vi "practica3.vi"() -> ()   [LabVIEW 2016]
uses:
  <vilib>/addons/Fuzzy Logic/NI_Fuzzy_Logic_API.lvlib
  <vilib>/addons/Fuzzy Logic/Membership/FL Create Membership Function (Trapezoid).vi
  <vilib>/addons/Fuzzy Logic/Membership/FL Create Membership Function (Triangle).vi
  <vilib>/addons/Fuzzy Logic/TypeDefs/FL Input_Output.ctl
  <vilib>/addons/Fuzzy Logic/TypeDefs/FL Modifier.ctl
panel:
  out "membership functions plot":cluster{cluster{"Xi":dbl, "Yi":dbl}[]}[](graph)
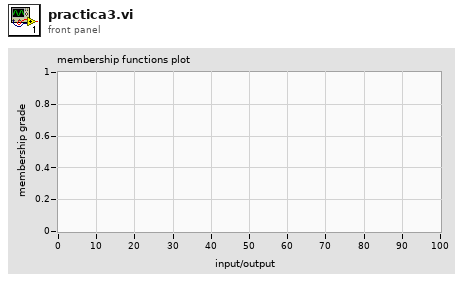
[diagram p1: front panel]
types:
  T1 = cluster{string, enum16{"triangular", "trapezoidal"}, dbl[]}[]
  T2 = typedef "NI_Fuzzy_Logic_API.lvlib/FL Input_Output.ctl" = u16
  T3 = typedef "NI_Fuzzy_Logic_API.lvlib/FL Modifier.ctl" = u16
  T4 = typedef "NI_Fuzzy_Logic_API.lvlib/FL Antecedent.ctl" = cluster{"Var Index":i32, "MF Index":i32, "Cond":T3}
  T5 = typedef "NI_Fuzzy_Logic_API.lvlib/FL Consequent.ctl" = cluster{"Var Index":i32, "MF Index":i32, "Cond":T3}
  T6 = typedef "NI_Fuzzy_Logic_API.lvlib/FL Membership Function.ctl" = cluster{"name":string, "shape":T7, "points":dbl[], "color":u32, "user-defined shape index":i32}
  T7 = typedef "NI_Fuzzy_Logic_API.lvlib/FL Membership Function Shape.ctl" = u16
  T8 = typedef "NI_Fuzzy_Logic_API.lvlib/FL Rule.ctl" = cluster{"antecedents":T4[], "antecedent connective":T9, "consequents":T5[], "consequent implication":T10, "degree of support":dbl}
  T9 = typedef "NI_Fuzzy_Logic_API.lvlib/FL Antecedent Connective.ctl" = u16
  T10 = typedef "NI_Fuzzy_Logic_API.lvlib/FL Consequent Implication.ctl" = u16
  T11 = typedef "NI_Fuzzy_Logic_API.lvlib/FL Variable.ctl" = cluster{"name":string, "range":dbl[], "MFs":T6[]}
  T12 = typedef "NI_Fuzzy_Logic_API.lvlib/FL System.ctl" = cluster{"input variables":T11[], "output variables":T11[], "rules":T8[], "defuzzification method":T13, "description":string, "user MF interpolating polynomials":T14[]}
  T13 = typedef "NI_Fuzzy_Logic_API.lvlib/FL Defuzzification.ctl" = u16
  T14 = typedef "NI_Fuzzy_Logic_API.lvlib/FL Interpolating polynomials.ctl" = cluster{"X":dbl[], "Y":dbl[], "Y(x) coeff":dbl[][], "X(y) coeff":dbl[][], "Area(y) coeff":dbl[][], "coa_x(y) coeff":dbl[][]}
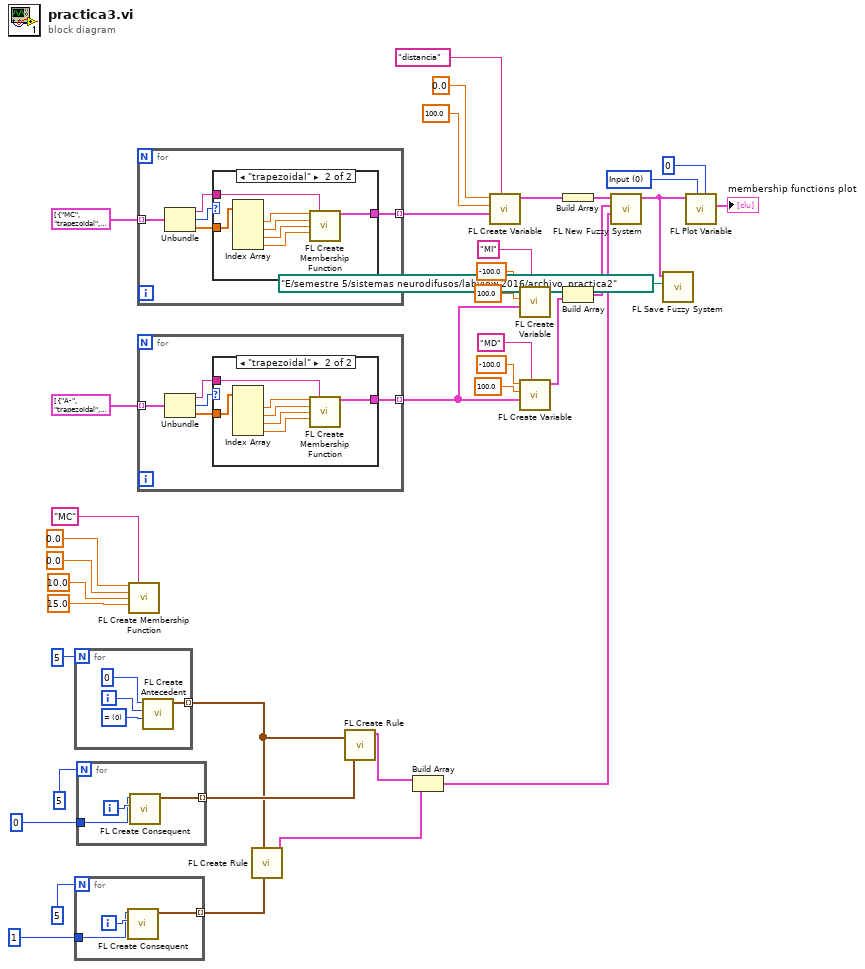
[diagram p0: block diagram]
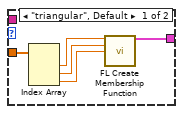
[diagram p2: hidden frame]
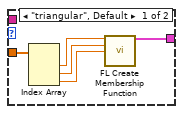
[diagram p3: hidden frame]
diagram:
  w26 = T2 0 items=["Input", "Output"] ("input/output")
  n1 = for {
    N: 5 -> [_]
    tunnel: [w40] -> w3 mode=indexing
    i -> [w43]
    w42 = T3 0 items=["=", "!="] ("condition")
    n2 = call <vilib>:"FL Create Antecedent.vi"("condition"=w42, "membership function index"=w43, "variable index"=0) -> ("antecedent"=w40:T4)  [unwired: 7 in, 1 out]
  }
  n3 = for {
    N: 5 -> [_]
    tunnel: [w45] -> w7 mode=indexing
    tunnel: 1 ("variable index") -> [w44]
    i -> [w46]
    n4 = call <vilib>:"FL Create Consequent.vi"("membership function index"=w46, "variable index"=w44) -> ("consequent"=w45:T5)  [unwired: 8 in, 1 out]
  }
  n5 = for {
    N: 5 -> [_]
    tunnel: [w48] -> w11 mode=indexing
    tunnel: 0 ("variable index") -> [w47]
    i -> [w49]
    n6 = call <vilib>:"FL Create Consequent.vi"("membership function index"=w49, "variable index"=w47) -> ("consequent"=w48:T5)  [unwired: 8 in, 1 out]
  }
  n7 = call-poly <vilib>:"FL Create Membership Function.vi"("left base"=0.0, "name"="MC", "left top"=0.0 ("top"), "right top"=10.0 ("right base"), "right base"=15.0) -> ()  [unwired: 9 in, 2 out]
  n8 = for {
    tunnel: T1 [{"MC", enum."trapezoidal", [0.0, 0.0, 10.0, 15.0]}, {"C", enum."triangular", [10.0, 25.0, 40.0]}, {"I", enum."triangular", [35.0, 50.0, 65.0]}, {"L", enum."triangular", [50.0, 75.0, 90.0]}, {"ML", enum."trapezoidal", [85.0, 90.0, 100.0, 100.0]}] -> [w54] mode=indexing
    tunnel: [w50] -> w30 mode=indexing
    n9 = Unbundle(w54) -> (w52:string, w53:enum16{"triangular", "trapezoidal"}, w51:dbl[])
    n10 = case shown="\"trapezoidal\"" w53 {
      tunnel: w52 -> [_ w66]
      tunnel: w51 -> [w59 w65]
      tunnel: [w55 w60] -> w50
      frame "triangular", Default {
        n11 = Index Array(array=w59) -> (element #1=w58:dbl, element #2=w57:dbl, element #3=w56:dbl)  [unwired: 3 in]
        n12 = call-poly <vilib>:"FL Create Membership Function.vi"("left base"=w58, "top"=w57, "right base"=w56) -> ("membership function"=w55:T6)  [unwired: 11 in, 1 out]
      }
      frame "trapezoidal" {
        n13 = Index Array(array=w65) -> (element #1=w64:dbl, element #2=w63:dbl, element #3=w62:dbl, element #4=w61:dbl)  [unwired: 4 in]
        n14 = call-poly <vilib>:"FL Create Membership Function.vi"("left base"=w64, "name"=w66, "left top"=w63, "right top"=w62, "right base"=w61) -> ("membership function"=w60:T6)  [unwired: 9 in, 1 out]
      }
    }
  }
  n15 = for {
    tunnel: T1 [{"A-", enum."trapezoidal", [-100.0, -100.0, -70.0, -50.0]}, {"M-", enum."triangular", [-70.0, -35.0, 0.0]}, {"Z", enum."triangular", [-10.0, 0.0, -10.0]}, {"M+", enum."triangular", [0.0, 35.0, 70.0]}, {"A+", enum."trapezoidal", [50.0, 70.0, 100.0, 100.0]}] -> [w71] mode=indexing
    tunnel: [w67] -> w17 mode=indexing
    n16 = Unbundle(w71) -> (w69:string, w70:enum16{"triangular", "trapezoidal"}, w68:dbl[])
    n17 = case shown="\"trapezoidal\"" w70 {
      tunnel: w69 -> [_ w83]
      tunnel: w68 -> [w76 w82]
      tunnel: [w72 w77] -> w67
      frame "triangular", Default {
        n18 = Index Array(array=w76) -> (element #1=w75:dbl, element #2=w74:dbl, element #3=w73:dbl)  [unwired: 3 in]
        n19 = call-poly <vilib>:"FL Create Membership Function.vi"("left base"=w75, "top"=w74, "right base"=w73) -> ("membership function"=w72:T6)  [unwired: 11 in, 1 out]
      }
      frame "trapezoidal" {
        n20 = Index Array(array=w82) -> (element #1=w81:dbl, element #2=w80:dbl, element #3=w79:dbl, element #4=w78:dbl)  [unwired: 4 in]
        n21 = call-poly <vilib>:"FL Create Membership Function.vi"("left base"=w81, "name"=w83, "left top"=w80, "right top"=w79, "right base"=w78) -> ("membership function"=w77:T6)  [unwired: 9 in, 1 out]
      }
    }
  }
  n22 = call <vilib>:"FL Create Rule.vi"("consequents"=w7, "antecedents"=w3) -> ("rule"=w6:T8)  [unwired: 8 in, 1 out]
  n23 = call <vilib>:"FL Create Rule.vi"("consequents"=w11, "antecedents"=w3) -> ("rule"=w5:T8)  [unwired: 8 in, 1 out]
  n24 = Build Array(w5, w6) -> (w4:T8[])
  n25 = call <vilib>:"FL Create Variable.vi"("name"="distancia", "membership functions"=w30, "maximum"=100.0, "minimum"=0.0) -> ("variable"=w27:T11)  [unwired: 6 in, 1 out]
  n26 = call <vilib>:"FL Create Variable.vi"("name"="MI", "membership functions"=w17, "maximum"=100.0, "minimum"=-100.0) -> ("variable"=w15:T11)  [unwired: 6 in, 1 out]
  n27 = call <vilib>:"FL Create Variable.vi"("name"="MD", "membership functions"=w17, "maximum"=100.0, "minimum"=-100.0) -> ("variable"=w16:T11)  [unwired: 6 in, 1 out]
  n28 = Build Array(w27) -> (w28:T11[])
  n29 = Build Array(w15, w16) -> (w14:T11[])
  n30 = call <vilib>:"FL New Fuzzy System.vi"("rules"=w4, "output variables"=w14, "input variables"=w28) -> ("fuzzy system out"=w2:T12)  [unwired: 7 in, 1 out]
  n31 = call <vilib>:"FL Save Fuzzy System.vi"("file path"=path "E:/semestre 5/sistemas neurodifusos/labview 2016/archivo_practica2", "fuzzy system in"=w2) -> ()  [unwired: 8 in, 2 out]
  n32 = call <vilib>:"FL Plot Variable.vi"("variable index"=0, "input/output"=w26, "fuzzy system in"=w2) -> ("membership functions plot"=→"membership functions plot":cluster{cluster{"Xi":dbl, "Yi":dbl}[]}[])  [unwired: 6 in, 2 out]
